vi "Store Configuration Parameters.vi"(8 "error in (no error)":errorcluster, 10 "refnum":T1, 11 "CompactDAQ Configuration in":refnum<class "CompactDAQ Configuration.lvclass">) -> (0 "error out":errorcluster, 2 "refnum out":T1, 3 "CompactDAQ Configuration out":refnum<class "CompactDAQ Configuration.lvclass">)   [LabVIEW 2017, in "CompactDAQ Configuration.lvclass"]
uses:
  CompactDAQ Configuration.lvclass
  <vilib>/Utility/config.llb/Config Data RefNum.ctl
  CompactDAQ Configuration.lvclass/CompactDAQ Configuration.ctl
  <userlib>/Common Components/Hardware/DAQ/config/DAQ Configuration.lvclass
  <vilib>/Utility/config.llb/NI_LVConfig.lvlib
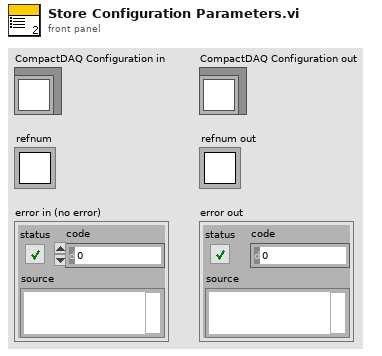
[diagram p1: front panel]
types:
  T1 = typedef "NI_LVConfig.lvlib/Config Data RefNum.ctl" = refnum<k1>
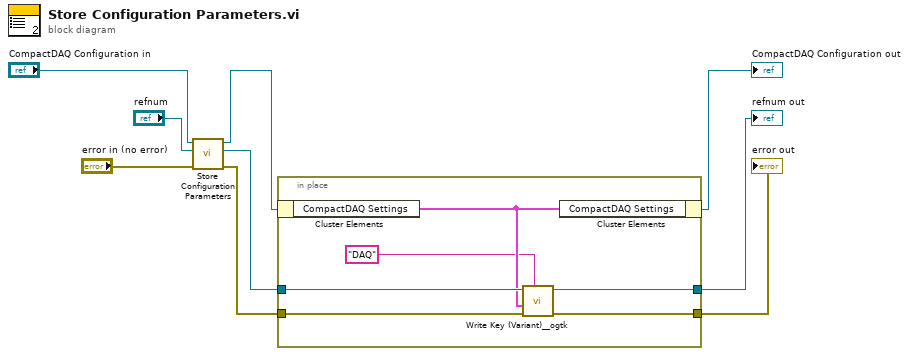
[diagram p0: block diagram]
diagram:
  n1 = call-parent "Store Configuration Parameters.vi"("error in (no error)"="error in (no error)", "refnum"="refnum", "DAQ Configuration in"="CompactDAQ Configuration in") -> ("error out"=w4:errorcluster, "refnum out"=w5:T1, "DAQ Configuration out"=w6:refnum<class "CompactDAQ Configuration.lvclass">)  [unwired: 6 in]
  n2 = in-place "In Place Element Structure" {
    in-place-border: w5 -> [w15]
    in-place-border: w4 -> [w14]
    in-place-border: [w11] -> w1
    in-place-border: [w10] -> w2
    n3 = in-place-cluster #1(w6) -> ("CompactDAQ Settings"=w13:cluster{"Allow Muxing?":bool})
    n4 = call <userlib>:"Write Key (Variant)__ogtk.vi"("section"="DAQ", "error in (no error)"=w14, "key-value"=w13, "refnum"=w15) -> ("error out"=w11:errorcluster, "refnum out"=w10:T1)  [unwired: 6 in]
    n5 = in-place-cluster #1("CompactDAQ Settings"=w13) -> (→"CompactDAQ Configuration out":refnum<class "CompactDAQ Configuration.lvclass">)
  }
  "error out" <- w1
  "refnum out" <- w2
